vi "Configure Reference Oscillator.vi"(8 "error in (no error)":errorcluster, 10 "Reference Oscillator (Internal)":enum16{"Internal", "External"}(ring), 11 "SA-FSW in":refnum<class "SA-FSW.lvclass">) -> (0 "error out":errorcluster, 3 "SA-FSW out":refnum<class "SA-FSW.lvclass">)   [LabVIEW 2020, in "SA-FSW.lvclass"]
uses:
  SA-FSW.lvclass
  C:/Sandbox/RF Bench/Source Code/WiSpry Test Framework/Instruments/Instrument.lvclass
  Instrument.lvclass/Instrument.ctl
  Instrument.lvclass
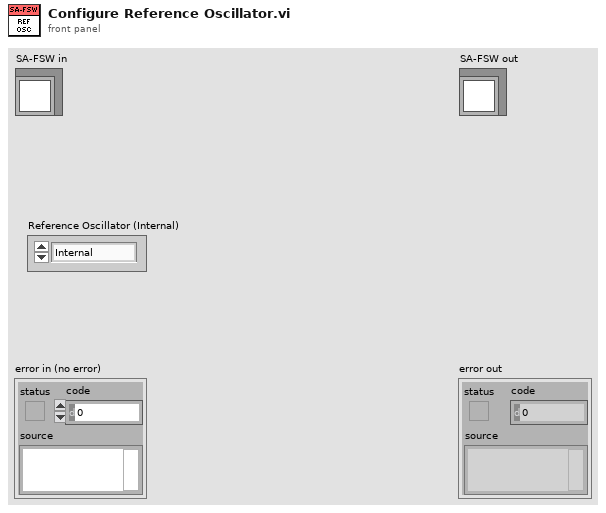
[diagram p1: front panel]
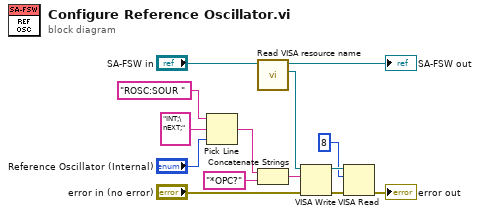
[diagram p0: block diagram]
diagram:
  n1 = Pick Line(string ("")="ROSC:SOUR ", multi-line string="INT;\nEXT;", line index="Reference Oscillator (Internal)") -> (output string=w10:string)
  n2 = call "Read VISA resource name.vi"("Instrument in"="SA-FSW in") -> ("VISA resource name"=w8:refnum<visa-resource-name>, "Instrument out"=→"SA-FSW out":refnum<class "SA-FSW.lvclass">)  [unwired: 9 in]
  n3 = Concatenate Strings(w10, "*OPC?" ("string")) -> (w6:string)
  n4 = VISA Write(VISA resource name=w8, write buffer=w6, error in (no error)="error in (no error)") -> (VISA resource name out=w4:refnum<visa-resource-name>, error out=w5:errorcluster)  [unwired: 1 out]
  n5 = VISA Read(VISA resource name=w4, byte count=u32 8, error in (no error)=w5) -> (error out=→"error out":errorcluster)  [unwired: 3 out]
